vi "DevControlPannel.vi"() -> ()   [LabVIEW 2017]
uses:
  C:/Code/CMCryoSysCode/Expose/COM/CSCom/CSCom/bin/Release/CSCom.dll
  Expose/COM/CSCom/CSCom/bin/Release/CSCom.dll
  <userlib>/_OpenG.lib/file/file.llb/File Exists - Scalar__ogtk.vi
  <vilib>/Utility/config.llb/Read Key (Path).vi
  <vilib>/Utility/config.llb/Write Key (Path).vi
  <vilib>/Utility/config.llb/NI_LVConfig.lvlib
panel:
  in  "Run on open":bool
  in  "btnOpenMatlabCode":bool
  in  "Search":string
  in  "btnOpenExperiment":bool
  in  "btnMakeTemplateFromExperiment":bool
  in  "Experiments":i32(listbox)
  in  "Current user path":path
  in  "btnExit":bool
  in  "btnLoadUserLib":bool
  in  "btnNewUserLib":bool
  in  "btnNewExperiment":bool
  # "Select an experiment to open, or make the experiment into a template. (User new experiment create from templates)."
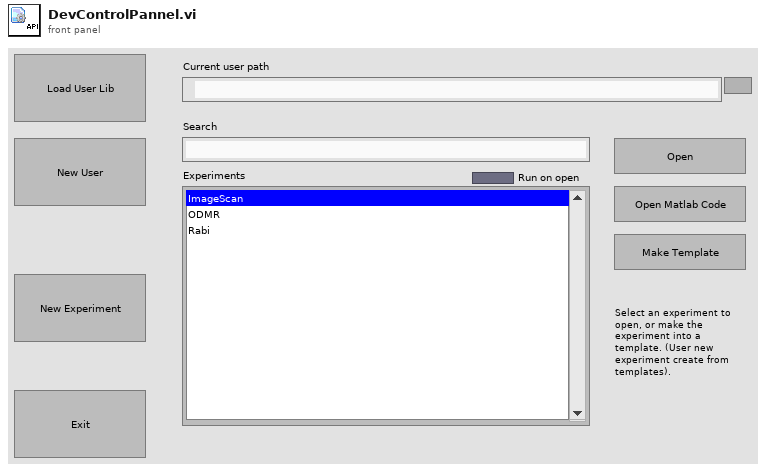
[diagram p1: front panel]
types:
  T1 = typedef "NI_LVConfig.lvlib/Config Data RefNum.ctl" = refnum<k1>
  T2 = typedef "ExposeEventRegistrationDataType.ctl" = refnum<event-registration>
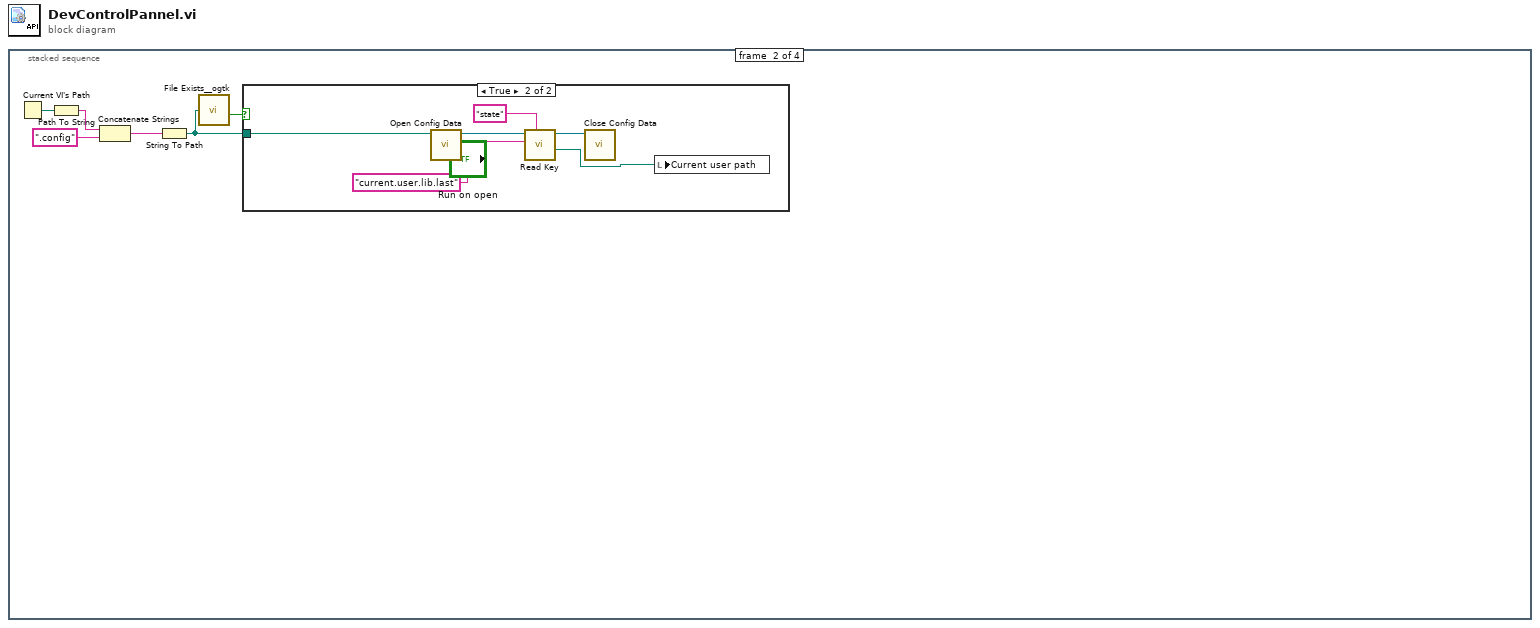
[diagram p0: block diagram]
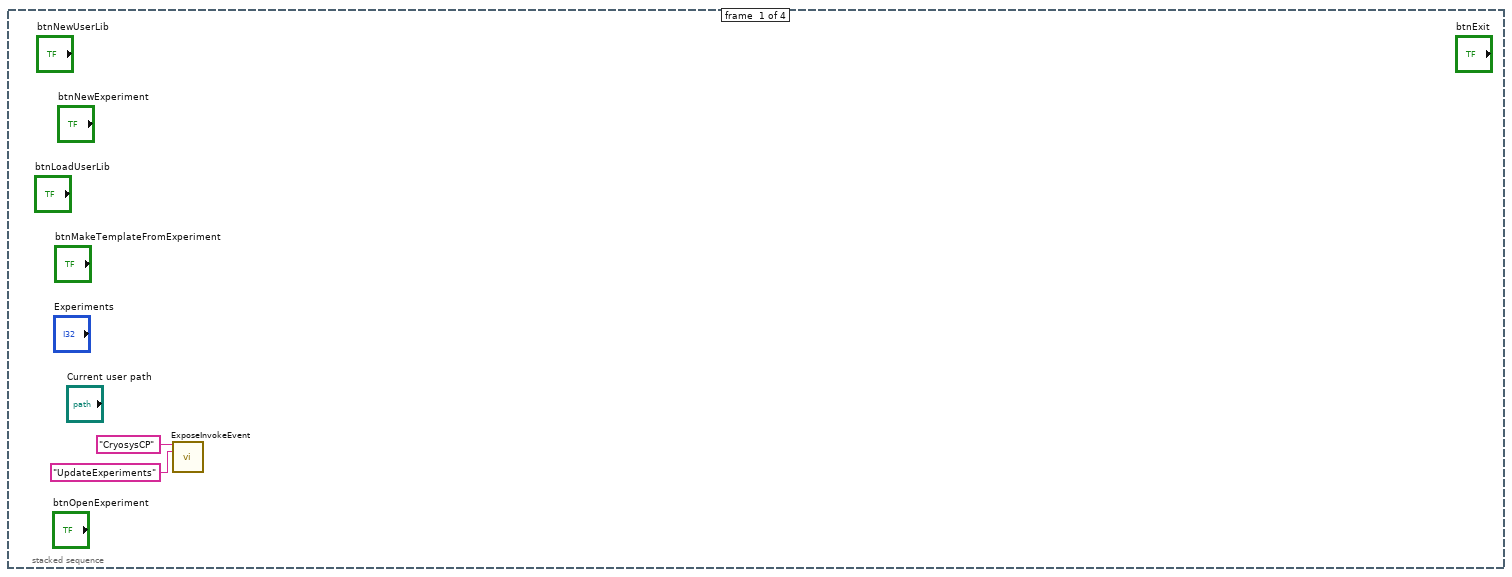
[diagram p2: hidden frame]
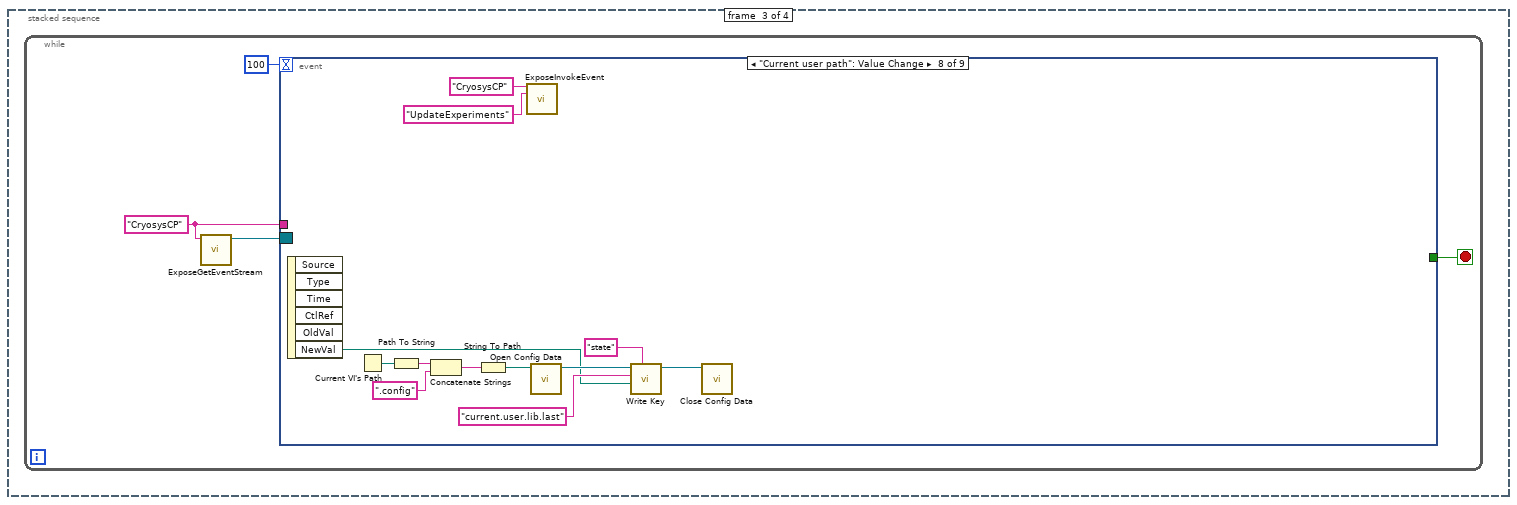
[diagram p4: hidden frame]
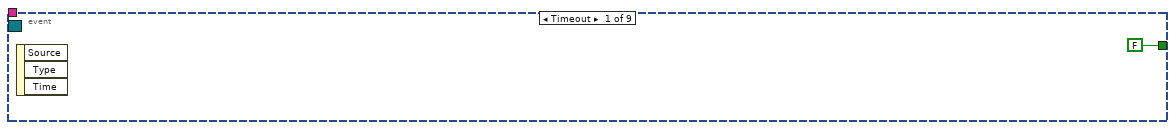
[diagram p5: hidden frame]
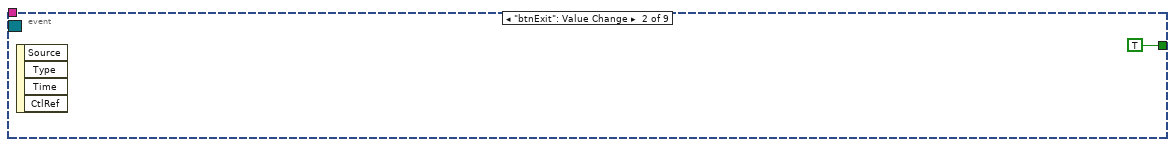
[diagram p6: hidden frame]
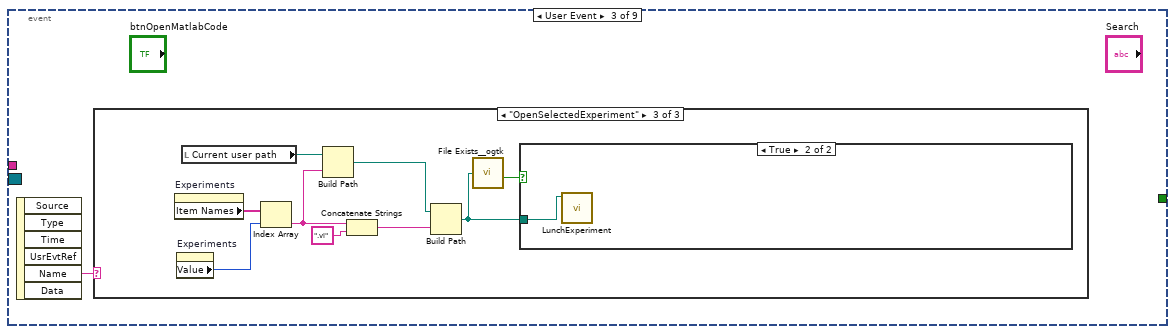
[diagram p7: hidden frame]
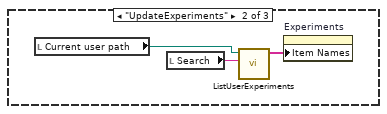
[diagram p9: hidden frame]
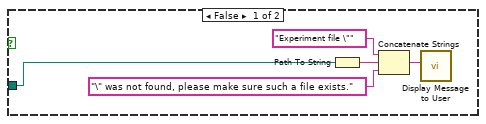
[diagram p10: hidden frame]
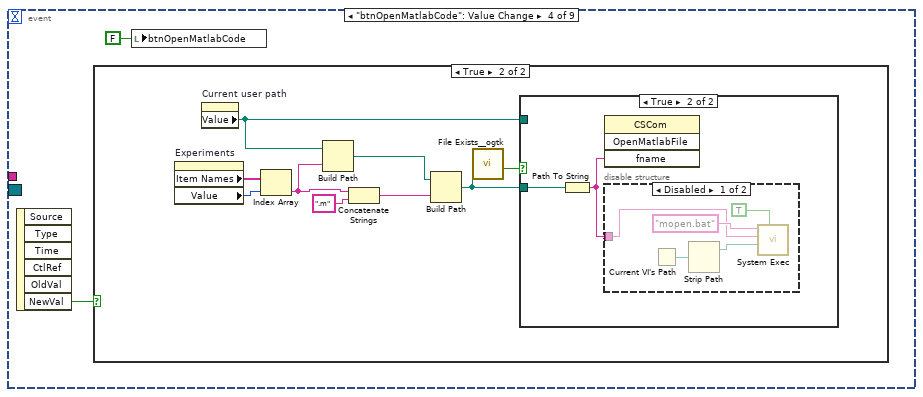
[diagram p11: hidden frame]
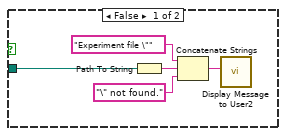
[diagram p13: hidden frame]
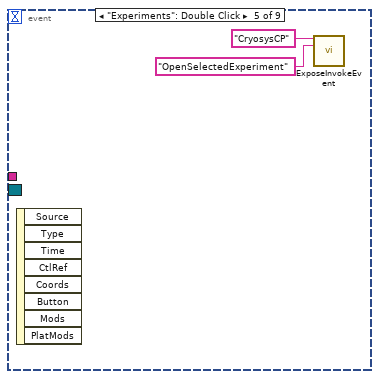
[diagram p15: hidden frame]
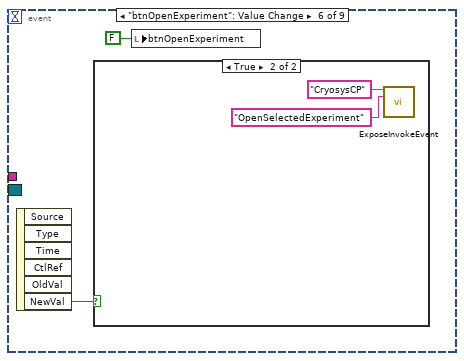
[diagram p16: hidden frame]
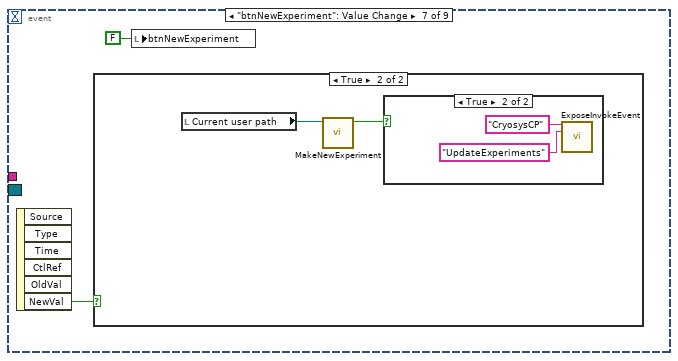
[diagram p18: hidden frame]
diagram:
  n1 = stacked-sequence {
    frame #0 {
      n2 = call "ExposeInvokeEvent.vi"("ID"="CryosysCP", "name"="UpdateExperiments") -> ()  [unwired: 13 in, 1 out]
    }
    frame #1 {
      n3 = Current VI's Path() -> (path=w7:path)
      n4 = Path To String(path=w7) -> (string=w6:string)
      n5 = Concatenate Strings(w6, ".config" ("name or relative path")) -> (w4:string)
      n6 = String To Path(string=w4) -> (path=w3:path)
      n7 = call-poly <userlib>:"File Exists__ogtk.vi"("file path"=w3) -> ("exists"=w8:bool)  [unwired: 6 in, 1 out]
      n8 = case shown="True" w8 {
        tunnel: w3 -> [_ w14]
        frame False {
        }
        frame True {
          n9 = call <vilib>:"Open Config Data.vi"("configuration file path"=w14) -> ("refnum"=w13:T1)  [unwired: 8 in, 2 out]
          n10 = call-poly <vilib>:"Read Key.vi"("section"="state", "key"="current.user.lib.last", "refnum"=w13) -> ("value"=w11:path, "refnum out"=w12:T1)  [unwired: 5 in, 2 out]
          n11 = call <vilib>:"Close Config Data.vi"("refnum"=w12) -> ()  [unwired: 9 in, 2 out]
          n12 = local write "Current user path"(w11) -> ()
        }
      }
    }
    frame #2 {
      n13 = while {
        stop <- w17 stop-if-true
        w16 = "CryosysCP" ("ID")
        n14 = call "ExposeGetEventStream.vi"("ID"=w16) -> ("Event Registration Refnum out"=w15:T2)  [unwired: 7 in, 3 out]
        n15 = event shown="[7] \"Current user path\": Value Change" {
          selector: w15 -> [_ _ _ _ _ _ _ _ _]
          dyn-events: _ -> [_ _ _ _ _ _ _ _ _]
          timeout: 100 -> [_ _ _ _ _ _ _ _ _]
          tunnel: [FALSE TRUE _ _ _ _ _ _ _] -> w17
          tunnel: w16 -> [_ _ _ _ _ _ _ _ _]
          event Timeout {
            n16 = event-data() -> ()  [unwired: 1 in, 3 out]
          }
          event "btnExit": Value Change {
            n17 = event-data() -> ()  [unwired: 1 in, 4 out]
          }
          event User Event {
            n18 = event-data() -> ("Name"=w21:string)  [unwired: 1 in, 5 out]
            n19 = case shown="\"OpenSelectedExperiment\"" w21 {
              frame Default {
              }
              frame "UpdateExperiments" {
                n20 = local read "Current user path"() -> (w22:path)
                n21 = local read "Search"() -> (w23:string)
                n22 = call "ListUserExperiments.vi"("Search"=w23, "Current user path"=w22) -> ("Sorted Array out"=w24:string[])  [unwired: 9 in]
                n23 = property on="Experiments" class="LstBox (strict)"("Item Names"=w24) -> ()  [unwired: 2 in, 2 out]
              }
              frame "OpenSelectedExperiment" {
                n24 = property on="Experiments" class="LstBox (strict)"() -> ("Item Names"=w33:string[])  [unwired: 2 in, 2 out]
                n25 = property on="Experiments" class="LstBox (strict)"() -> ("Value"=w32:i32)  [unwired: 2 in, 2 out]
                n26 = local read "Current user path"() -> (w31:path)
                n27 = Index Array(array=w33, index=w32) -> (element=w30:string)
                n28 = Build Path(base path=w31, name or relative path=w30) -> (appended path=w28:path)
                n29 = Concatenate Strings(w30, ".vi" ("string")) -> (w29:string)
                n30 = Build Path(base path=w28, name or relative path=w29) -> (appended path=w26:path)
                n31 = call-poly <userlib>:"File Exists__ogtk.vi"("file path"=w26) -> ("exists"=w27:bool)  [unwired: 6 in, 1 out]
                n32 = case shown="True" w27 {
                  tunnel: w26 -> [w36 w39]
                  frame False {
                    n33 = Path To String(path=w36) -> (string=w35:string)
                    n34 = Concatenate Strings("Experiment file \"" ("string"), w35, "\" was not found, please make sure such a file exists." ("string")) -> (w34:string)
                    n35 = call "Display Message to User"("Message"=w34) -> ()  [unwired: 9 in, 2 out]
                  }
                  frame True {
                    n36 = call "LunchExperiment.vi"("appended path"=w39) -> ()  [unwired: 11 in]
                  }
                }
              }
            }
          }
          event "btnOpenMatlabCode": Value Change {
            n37 = event-data() -> ("NewVal"=w40:bool)  [unwired: 1 in, 5 out]
            n38 = case shown="True" w40 {
              frame False {
              }
              frame True {
                n39 = property on="Experiments" class="LstBox (strict)"() -> ("Item Names"=w50:string[], "Value"=w49:i32)  [unwired: 2 in, 2 out]
                n40 = property on="Current user path" class="Path"() -> ("Value"=w42:path)  [unwired: 2 in, 2 out]
                n41 = Index Array(array=w50, index=w49) -> (element=w47:string)
                n42 = Build Path(base path=w42, name or relative path=w47) -> (appended path=w48:path)
                n43 = Concatenate Strings(w47, ".m" ("string")) -> (w45:string)
                n44 = Build Path(base path=w48, name or relative path=w45) -> (appended path=w43:path)
                n45 = call-poly <userlib>:"File Exists__ogtk.vi"("file path"=w43) -> ("exists"=w44:bool)  [unwired: 6 in, 1 out]
                n46 = case shown="True" w44 {
                  tunnel: w43 -> [w51 w57]
                  tunnel: w42 -> [_ _]
                  frame False {
                    n47 = Path To String(path=w51) -> (string=w53:string)
                    n48 = Concatenate Strings("Experiment file \"" ("string"), w53, "\" not found." ("string")) -> (w52:string)
                    n49 = call "Display Message to User2"("Message"=w52) -> ()  [unwired: 9 in, 2 out]
                  }
                  frame True {
                    n50 = Path To String(path=w57) -> (string=w56:string)
                    n51 = invoke class="CSCom" method="OpenMatlabFile"("fname"=w56) -> ()  [unwired: 3 in, 4 out]
                    n52 = disable-structure shown="Disabled" {
                      disable-tunnel: w56 -> [w58 _]
                      frame Disabled {
                        n53 = Current VI's Path() -> (path=w61:path)
                        n54 = Strip Path(path=w61) -> (stripped path=w60:path)  [unwired: 1 out]
                        n55 = call <vilib>:"System Exec.vi"("wait until completion? (T)"=TRUE, "working directory"=w60, "standard input"=w58, "command line"="mopen.bat") -> ()  [unwired: 4 in, 4 out]
                      }
                      frame Enabled {
                      }
                    }
                  }
                }
              }
            }
            n56 = local write "btnOpenMatlabCode"(FALSE ("btnOpenMatlabCode")) -> ()
          }
          event "Experiments": Double Click {
            n57 = event-data() -> ()  [unwired: 1 in, 8 out]
            n58 = call "ExposeInvokeEvent.vi"("ID"="CryosysCP", "name"="OpenSelectedExperiment") -> ()  [unwired: 13 in, 1 out]
          }
          event "btnOpenExperiment": Value Change {
            n59 = event-data() -> ("NewVal"=w66:bool)  [unwired: 1 in, 5 out]
            n60 = case shown="True" w66 {
              frame False {
              }
              frame True {
                n61 = call "ExposeInvokeEvent.vi"("ID"="CryosysCP", "name"="OpenSelectedExperiment") -> ()  [unwired: 13 in, 1 out]
              }
            }
            n62 = local write "btnOpenExperiment"(FALSE ("btnOpenExperiment")) -> ()
          }
          event "btnNewExperiment": Value Change {
            n63 = event-data() -> ("NewVal"=w70:bool)  [unwired: 1 in, 5 out]
            n64 = case shown="True" w70 {
              frame False {
              }
              frame True {
                n65 = local read "Current user path"() -> (w72:path)
                n66 = call "MakeNewExperiment.vi"("User Libraray in"=w72) -> ("Created OK"=w71:bool)  [unwired: 9 in, 1 out]
                n67 = case shown="True" w71 {
                  frame False {
                  }
                  frame True {
                    n68 = call "ExposeInvokeEvent.vi"("ID"="CryosysCP", "name"="UpdateExperiments") -> ()  [unwired: 13 in, 1 out]
                  }
                }
              }
            }
            n69 = local write "btnNewExperiment"(FALSE ("btnNewExperiment")) -> ()
          }
          event "Current user path": Value Change {
            n70 = event-data() -> ("NewVal"=w82:path)  [unwired: 1 in, 5 out]
            n71 = Current VI's Path() -> (path=w79:path)
            n72 = Path To String(path=w79) -> (string=w78:string)
            n73 = Concatenate Strings(w78, ".config" ("name or relative path")) -> (w76:string)
            n74 = String To Path(string=w76) -> (path=w75:path)
            n75 = call "ExposeInvokeEvent.vi"("ID"="CryosysCP", "name"="UpdateExperiments") -> ()  [unwired: 13 in, 1 out]
            n76 = call <vilib>:"Open Config Data.vi"("configuration file path"=w75) -> ("refnum"=w84:T1)  [unwired: 8 in, 2 out]
            n77 = call-poly <vilib>:"Write Key.vi"("section"="state", "value"=w82, "key"="current.user.lib.last", "refnum"=w84) -> ("refnum out"=w81:T1)  [unwired: 5 in, 2 out]
            n78 = call <vilib>:"Close Config Data.vi"("refnum"=w81) -> ()  [unwired: 9 in, 2 out]
          }
          event "Search": Value Change {
            n79 = event-data() -> ()  [unwired: 1 in, 6 out]
            n80 = call "ExposeInvokeEvent.vi"("ID"="CryosysCP", "name"="UpdateExperiments") -> ()  [unwired: 13 in, 1 out]
          }
        }
      }
    }
    frame #3 {
      n81 = control-ref of="This VI"() -> (w89:refnum<vi>)
      n82 = invoke class="VI" method="FP.Close"(reference=w89) -> ()  [unwired: 2 in, 3 out]
    }
  }
